vi "Vision Research Phantom Series PhCon PhNVMRestore.vi"(0 "CN in":u32=1, 1 "CineNo":u32, 5 "Error In (no error)":errorcluster, 7 "CallID":u32) -> (14 "CN out":u32=1, 19 "Error Out":errorcluster)   [LabVIEW 2013, in "VRI.lvlib"]
doc: "PhCon.dll\n\nPhNVMRestore\nHRESULT PhNVMRestore(UINT CN, int Cine, UINT CallID);\n\nParameters Description\nCN (in) Camera number\nCineNo (in) Cine number\nCallID (in) Callback function to see the progress\nReturn HRESULT (0=Ok)\nComments Transfer the specified cine from the NVMemory to DRAM.\n Only for v4...v6. In v7 NVM cines can be read the same \n way as FBM cines.\n\nWritten by:\nBLOOMY CONTROLS, INC\nWINDSOR, CT 06095, USA\n860-298-9925\nwww.bloomy.com\nV1.0.0\nMay, 2004"
uses:
  VRI.lvlib
  Phantom DLLs/PhCon.dll
panel:
  # "For instructions on the use of this VI, press Ctrl+H to display the help window and move the mouse over the icon, controls, and indicators"
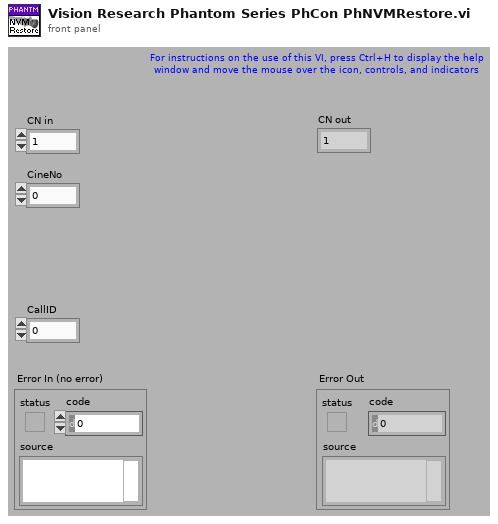
[diagram p1: front panel]
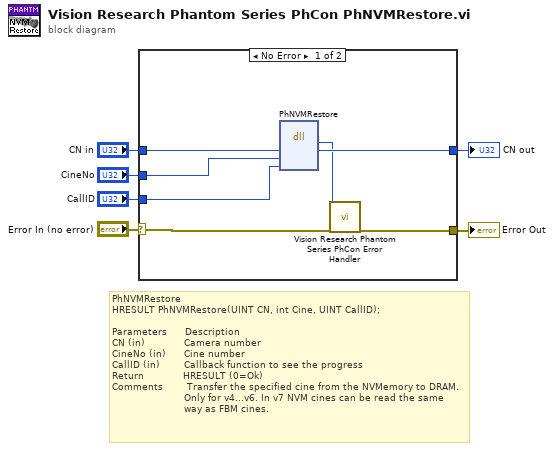
[diagram p0: block diagram]
diagram:
  # "PhNVMRestore\nHRESULT PhNVMRestore(UINT CN, int Cine, UINT CallID);\n\nParameters      Description\nCN (in)             Camera number\nCineNo (in)      Cine number\nCallID (in)        Callback function to see the progress\nReturn             HRESULT (0=Ok)\nComments        Transfer the specified cine from the NVMemory to DRAM.\n                        Only for v4...v6. In v7 NVM cines can be read the same \n                        way as FBM cines."
  n1 = case shown="No Error" "Error In (no error)" {
    selector: "Error In (no error)" -> [w13 w14]
    tunnel: [w12 w14] -> w5
    tunnel: "CN in" -> [w11 _]
    tunnel: [w10 _] -> w3
    tunnel: "CallID" -> [w9 _]
    tunnel: "CineNo" -> [w8 _]
    frame No Error {
      n2 = dll-call lib="C:/Projects/SDK/32-bit/Vision Research Phantom Series Labview Driver/Phantom DLLs/PhCon.dll" fn="PhNVMRestore"("CN"=w11, "CineNo"=w8, "CallID"=w9) -> ("HRESULT"=w7:i32, "CN"=w10:u32)  [unwired: 5 in, 2 out]
      n3 = call "Vision Research Phantom Series PhCon Error Handler.vi"("ErrNo"=w7, "Error In (no error)"=w13) -> ("Error Out"=w12:errorcluster)  [unwired: 17 out]
    }
    frame Error {
    }
  }
  "Error Out" <- w5
  "CN out" <- w3
